vi "Modbus_Pid_Control.vi"(6 "register values":u16[](array[numeric]), 9 "new D":dbl, 10 "new I":dbl, 11 "new P":dbl) -> (1 "Numeric":dbl, 2 "Numeric 2":dbl, 3 "Numeric 3":dbl, 4 "Boolean":bool)   [LabVIEW 2020]
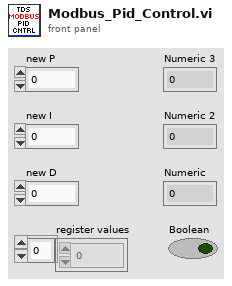
[diagram p1: front panel]
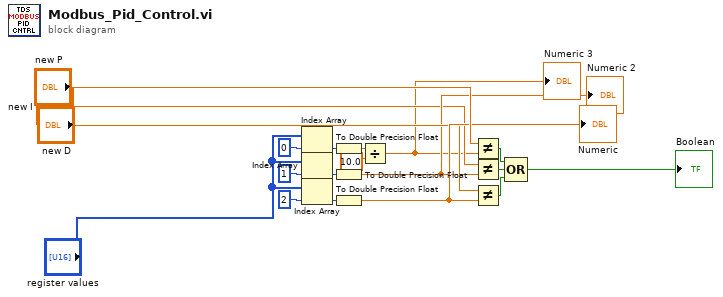
[diagram p0: block diagram]
diagram:
  n1 = Index Array(array="register values", index=0) -> (element=w7:u16)
  n2 = Index Array(array="register values", index=1) -> (element=w6:u16)
  n3 = Index Array(array="register values", index=2) -> (element=w5:u16)
  n4 = To Double Precision Float(number=w7) -> (double precision float=w8:dbl)
  n5 = To Double Precision Float(number=w6) -> (double precision float=w11:dbl)
  "Numeric 2" <- w11
  n6 = To Double Precision Float(number=w5) -> (double precision float=w13:dbl)
  "Numeric" <- w13
  n7 = Divide(x=w8, y=10.0) -> (x/y=w9:dbl)
  "Numeric 3" <- w9
  n8 = Not Equal?(x="new P", y=w9) -> (x != y?=w14:bool)
  n9 = Not Equal?(x="new I", y=w11) -> (x != y?=w15:bool)
  n10 = Not Equal?(x="new D", y=w13) -> (x != y?=w16:bool)
  n11 = Compound Arithmetic op=OR(w14, w15, w16) -> (→"Boolean":bool)
